vi "PCO_SetInterfaceOutputFormat.vi"(8 "error in (no error)":errorcluster {"code" format="%x"}, 9 "wFormat":u16(ring) items=["SCCMOS_FORMAT_TOP_BOTTOM"=0, "SCCMOS_FORMAT_TOP_CENTER_BOTTOM_CENTER"=256, "SCCMOS_FORMAT_CENTER_TOP_CENTER_BOTTOM"=512, "SCCMOS_FORMAT_CENTER_TOP_BOTTOM_CENTER"=768, "SCCMOS_FORMAT_TOP_CENTER_CENTER_BOTTOM"=1024], 10 "wDestInterface":u16(ring)=2 items=["edge"=2], 11 "ph":u64) -> (0 "error out":errorcluster {"code" format="%x"}, 2 "ErrorMessage":i32 format="%x", 3 "ph out":u64)   [LabVIEW 2019, in "SDK.lvlib" / "SpecialCommandsEdge.lvlib"]
doc: "<b>Description:</b>\nThis function does set the current interface output format.\nThe interface output format reflects the currently SCCMOS Readout Format of the camera.\nWith the SCCMOS Readout Format the data readout direction of the camera can be controlled.\nFor all cameras with Camera Link interface it is recommended to use PCO_SetTransferParameter function instead of this function, because the driver layer must be informed about any changes in readout format to successfully rearrange the image data.\n\n<b>Supported camera type:</b>\npco.edge\n\n<b>Descriptor dependency:</b>\nNone"
uses:
  SpecialCommandsEdge.lvlib
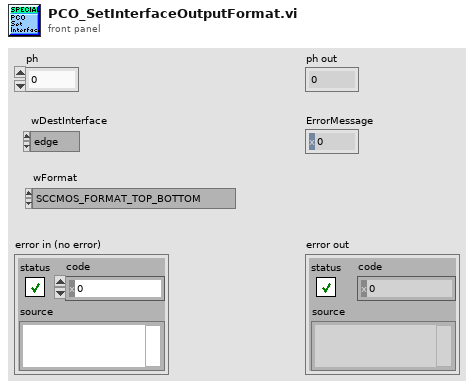
[diagram p1: front panel]
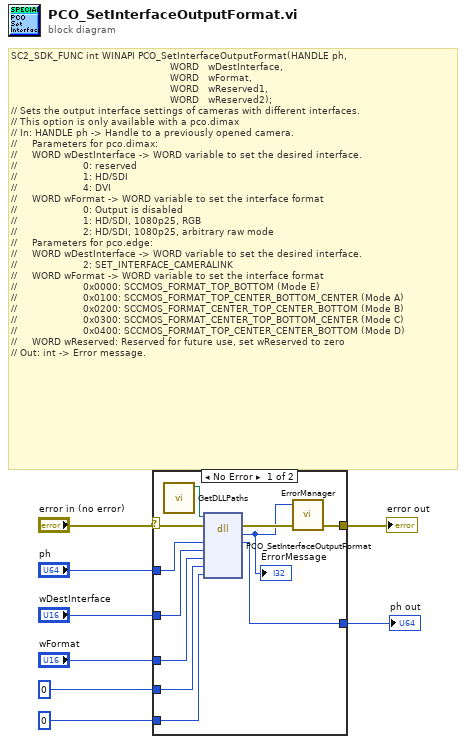
[diagram p0: block diagram]
diagram:
  # "SC2_SDK_FUNC int WINAPI PCO_SetInterfaceOutputFormat(HANDLE ph,\n                                                     WORD   wDestInterface,\n                                                     WORD   wFormat,\n                                                     WORD   wReserved1,\n                                                     WORD   wReserved2);\n// Sets the output interface settings of cameras with different interfaces.\n// This option is only available with a pco.dimax\n// In: HANDLE ph -> Handle to a previously opened camera.\n//     Parameters for pco.dimax:\n//     WORD wDestInterface -> WORD variable to set the desired interface.\n//                      0: reserved\n//                      1: HD/SDI\n//                      4: DVI\n//     WORD wFormat -> WORD variable to set the interface format\n//                      0: Output is disabled\n//                      1: HD/SDI, 1080p25, RGB\n//                      2: HD/SDI, 1080p25, arbitrary raw mode\n//     Parameters for pco.edge:\n//     WORD wDestInterface -> WORD variable to set the desired interface.\n//                      2: SET_INTERFACE_CAMERALINK\n//     WORD wFormat -> WORD variable to set the interface format\n//                      0x0000: SCCMOS_FORMAT_TOP_BOTTOM (Mode E)\n//                      0x0100: SCCMOS_FORMAT_TOP_CENTER_BOTTOM_CENTER (Mode A)\n//                      0x0200: SCCMOS_FORMAT_CENTER_TOP_CENTER_BOTTOM (Mode B)\n//                      0x0300: SCCMOS_FORMAT_CENTER_TOP_BOTTOM_CENTER (Mode C)\n//                      0x0400: SCCMOS_FORMAT_TOP_CENTER_CENTER_BOTTOM (Mode D)\n//     WORD wReserved: Reserved for future use, set wReserved to zero\n// Out: int -> Error message."
  n1 = case shown="No Error" "error in (no error)" {
    selector: "error in (no error)" -> [w13 w21]
    tunnel: "ph" -> [w19 w20]
    tunnel: [w18 w20] -> w7
    tunnel: [w11 w21] -> w6
    tunnel: u16 0 -> [w17 _]
    tunnel: "wFormat" -> [w16 _]
    tunnel: "wDestInterface" -> [w15 _]
    tunnel: u16 0 -> [w14 _]
    frame No Error {
      n2 = call "GetDLLPaths.vi"() -> ("SC2_Cam_Path"=w9:path)  [unwired: 9 in, 2 out]
      n3 = dll-call lib="?" fn="PCO_SetInterfaceOutputFormat"(path in=w9, error in=w13, "ph"=w19, "wDestInterface"=w15, "wFormat"=w16, "wReserved1"=w14, "wReserved2"=w17) -> (error out=w12:errorcluster, "return type"=w10:i32, "ph"=w18:u64)  [unwired: 5 in, 1 out]
      "ErrorMessage" <- w10
      n4 = call "ErrorManager.vi"("error in (no error)"=w12, "error code"=w10) -> ("error out"=w11:errorcluster)  [unwired: 3 in]
    }
    frame Error {
    }
  }
  "ph out" <- w7
  "error out" <- w6
